vi "GetStringPropertyValueInArray.vi"(0 "Array In":refnum<k24>[](array[refnum])) -> (1 "Array Out":refnum<k24>[](array[refnum]), 2 "String Value Property":string, 3 "error out":errorcluster)   [LabVIEW 2011]
uses:
  D:/tsdev/Tests/LVBuildValidation/11.0/Automated/FlexLVAdapter30/Refnums/DotNetRefnum/LabviewDNTest.dll
  LabviewDNTest.dll
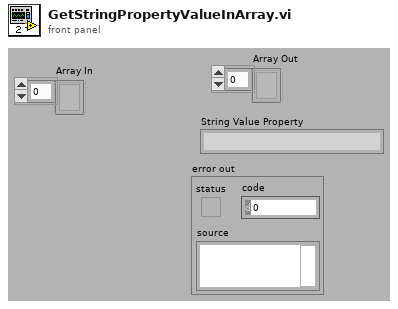
[diagram p1: front panel]
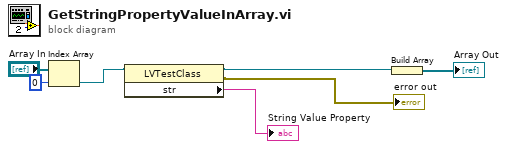
[diagram p0: block diagram]
diagram:
  n1 = Index Array(array="Array In", index=0) -> (element=w4:refnum<k24>)
  n2 = property class="LVTestClass"(reference=w4) -> (reference out=w3:refnum<k24>, error out=→"error out":errorcluster, "str"=→"String Value Property":string)  [unwired: 1 in]
  n3 = Build Array(w3) -> (→"Array Out":refnum<k24>[])
